vi "getListBoxRowIndex.vi"(8 "error in (no error)":errorcluster, 11 "ScriptEditorV2 in":refnum<class "ScriptEditorV2.lvclass">) -> (0 "error out":errorcluster, 2 "rowIndex":i32, 3 "ScriptEditorV2 out":refnum<class "ScriptEditorV2.lvclass">)   [LabVIEW 2009, in "Views.lvlib" / "ScriptEditor.lvlib" / "ScriptEditorV2.lvclass"]
uses:
  ScriptEditorV2.lvclass
  ScriptEditorV2.lvclass/ScriptEditorV2.ctl
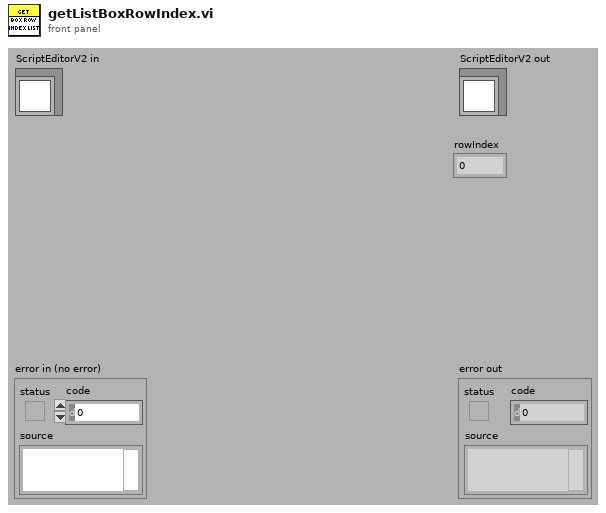
[diagram p1: front panel]
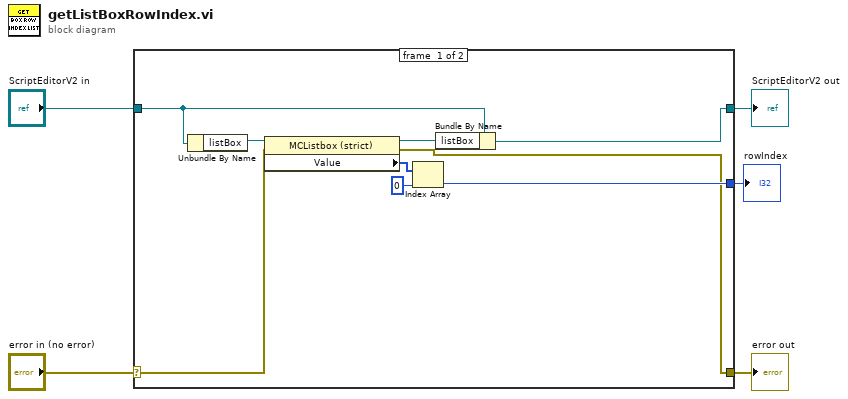
[diagram p0: block diagram]
diagram:
  n1 = case shown="No Error" "error in (no error)" {
    selector: "error in (no error)" -> [w7 w16]
    tunnel: [w6 w16] -> w4
    tunnel: [w9 w15] -> w2
    tunnel: "ScriptEditorV2 in" -> [w10 w15]
    tunnel: [w8 _] -> w1
    frame #0 {
      n2 = Unbundle By Name(w10) -> ("listBox"=w14:refnum<vi>)
      n3 = property class="MCListbox (strict)"(reference=w14, error in=w7) -> (reference out=w13:refnum<vi>, error out=w6:errorcluster, "Value"=w12:i32[])
      n4 = Index Array(array=w12, index=0) -> (element=w8:i32)
      n5 = Bundle By Name(cluster=w10, "listBox"=w13) -> (w9:refnum<class "ScriptEditorV2.lvclass">)
    }
    frame #1 {
    }
  }
  "error out" <- w4
  "ScriptEditorV2 out" <- w2
  "rowIndex" <- w1
